vi "Calcualte General Tardiness.vi"(9 "Due Dates":u16[](array[numeric]), 11 "Job Completion Times":u16[](array[numeric])) -> (3 "Total Tardiness (U16)":u16)   [LabVIEW 2013]
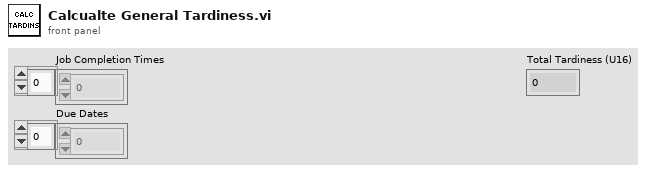
[diagram p1: front panel]
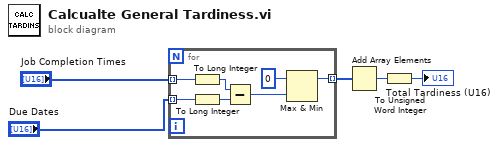
[diagram p0: block diagram]
diagram:
  n1 = for {
    tunnel: "Job Completion Times" -> [w9] mode=indexing
    tunnel: "Due Dates" -> [w8] mode=indexing
    tunnel: [w10] -> w2 mode=indexing
    n2 = To Long Integer(number=w9) -> (32bit integer=w6:i32)
    n3 = To Long Integer(number=w8) -> (32bit integer=w7:i32)
    n4 = Subtract(x=w6, y=w7) -> (x-y=w12:i32)
    n5 = Max & Min(x=0, y=w12) -> (max(x,y)=w10:i32)  [unwired: 1 out]
  }
  n6 = Add Array Elements(numeric array=w2) -> (sum=w1:i32)
  n7 = To Unsigned Word Integer(number=w1) -> (unsigned 16bit integer=→"Total Tardiness (U16)":u16)
